vi "Control Loop (Set).vi"(6 "ISOBUS address":T4=-1 caption="ISOBUS address (-1)", 8 "error in":errorcluster, 10 "Control Loop":T3, 11 "Mercury Reference In":T5) -> (0 "error out":errorcluster, 2 "Response":T1, 3 "Mercury Reference Out":T5, 4 "Valid?":T2)   [LabVIEW 2014, in "Mercury iXX.lvlib" / "Control Loop.lvlib"]
doc: "Set the control loop values."
uses:
  Control Loop.lvlib
  Controls/Mercury Reference.ctl
  Controls/Comms Transport Layer.ctl
  Private/Controls/Query Dynamic Reference.ctl
  Controls/ISOBus Address.ctl
  Temperature/Controls/Loop Cluster.ctl
  Controls/Is Valid LED.ctl
  Controls/Response String.ctl
  Private/Controls/Command Verbs.ctl
  Mercury iXX.lvlib
  Temperature.lvlib
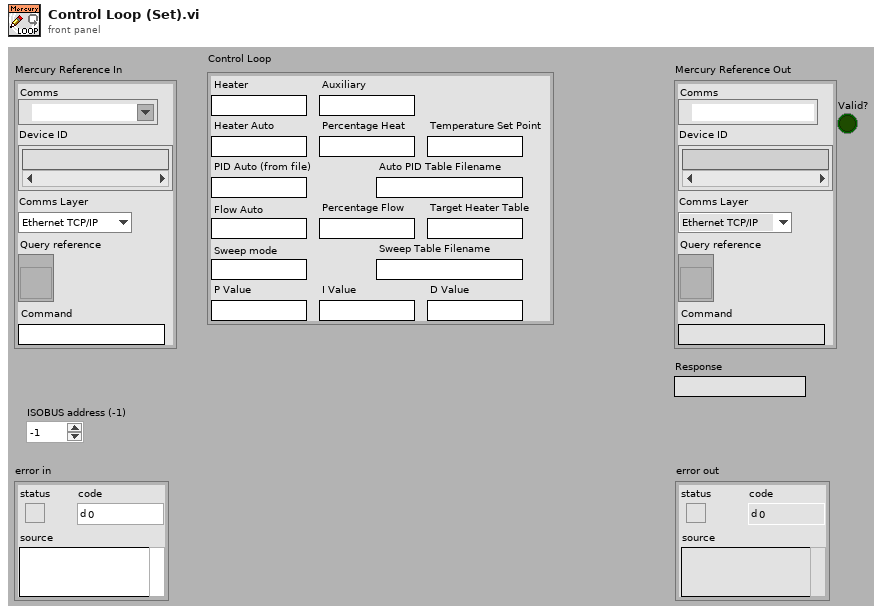
[diagram p1: front panel]
types:
  T1 = typedef "Mercury iXX.lvlib/Response String.ctl" = string
  T2 = typedef "Mercury iXX.lvlib/Is Valid LED.ctl" = bool
  T3 = typedef "Mercury iXX.lvlib/Temperature.lvlib/Loop Cluster.ctl" = cluster{"Heater":string, "Auxiliary":string, "Heater Auto":string, "Percentage Heat":string, "Temperature Set Point":string, "PID Auto (from file)":string, "P Value":string, "I Value":string, "D Value":string, "Auto PID Table Filename":string, "Flow Auto":string, "Target Heater Table":string, "Sweep mode":string, "Sweep Table Filename":string, "Percentage Flow":string}
  T4 = typedef "Mercury iXX.lvlib/ISOBus Address.ctl" = i32
  T5 = typedef "Mercury iXX.lvlib/Mercury Reference.ctl" = cluster{"Comms":refnum<visa-resource-name>, "Device ID":string[], "Comms Layer":T6, "Command":string, "Query reference":T7}
  T6 = typedef "Mercury iXX.lvlib/Comms Transport Layer.ctl" = enum16{"Ethernet TCP/IP", "USB", "ISOBus - RS-232", "GPIB"}
  T7 = typedef "Mercury iXX.lvlib/Query Dynamic Reference.ctl" = refnum<vi>
  T8 = typedef "Mercury iXX.lvlib/Command Verbs.ctl" = string
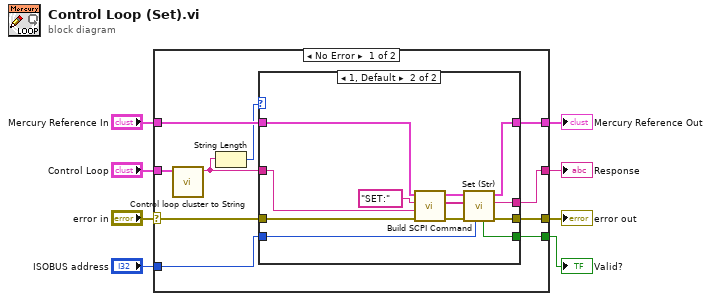
[diagram p0: block diagram]
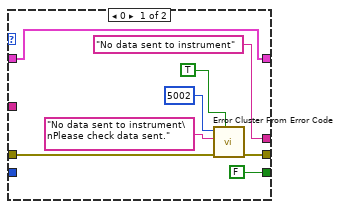
[diagram p2: hidden frame]
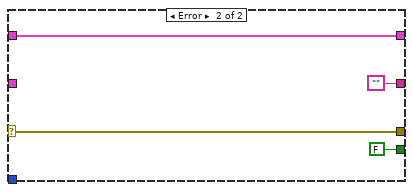
[diagram p3: hidden frame]
diagram:
  n1 = case shown="No Error" "error in" {
    selector: "error in" -> [w16 w41]
    tunnel: "Mercury Reference In" -> [w18 w42]
    tunnel: [w14 w42] -> w7
    tunnel: [w15 w41] -> w6
    tunnel: "ISOBUS address" -> [w17 _]
    tunnel: [w9 ""] -> w2
    tunnel: [w10 FALSE ("Valid?")] -> w3
    tunnel: "Control Loop" -> [w11 _]
    frame No Error {
      n2 = call "Control loop cluster to String.vi"("Control Loop"=w11) -> ("Data to send"=w12:string)  [unwired: 1 in, 9 out]
      n3 = String Length(string=w12) -> (length=w13:i32)
      n4 = case shown="1, Default" w13 {
        tunnel: w18 -> [w26 w27]
        tunnel: w17 -> [_ w31]
        tunnel: w16 -> [w24 w33]
        tunnel: [w25 w32] -> w15
        tunnel: [w26 w28] -> w14
        tunnel: w12 -> [_ w34]
        tunnel: [T2 FALSE ("Valid?") w30] -> w10
        tunnel: ["No data sent to instrument" ("Data") w29] -> w9
        frame 0 {
          n5 = call <vilib>:"Error Cluster From Error Code.vi"("show call chain? (False)"=TRUE, "error in (no error)"=w24, "error message (\"\")"="No data sent to instrument\nPlease check data sent." ("error message (\"\")"), "error code (0)"=5002) -> ("error out"=w25:errorcluster)  [unwired: 5 out]
        }
        frame 1, Default {
          n6 = call "Build SCPI Command.vi"("error in"=w33, "Noun(s)"=w34, "Verb"=T8 "SET:", "Mercury Reference In"=w27) -> ("error out"=w38:errorcluster, "SCPI Message(s)"=w37:string[], "Mercury Reference Out"=w36:T5)  [unwired: 5 out]
          n7 = call "Set (Str).vi"("ISOBUS address"=w31, "error in"=w38, "SCPI Message(s)"=w37, "Mercury Reference In"=w36) -> ("error out"=w32:errorcluster, "Response"=w29:T1, "Mercury Reference Out"=w28:T5, "Valid?"=w30:T2)  [unwired: 1 in, 3 out]
        }
      }
    }
    frame Error {
    }
  }
  "Mercury Reference Out" <- w7
  "error out" <- w6
  "Valid?" <- w3
  "Response" <- w2
